vi "Manager QueryPlugin.vi"(6 "contextId":T1, 8 "error in":errorcluster, 9 "timeout (ms)":i32=-1, 10 "Request Data":T17, 11 "gRPC ID":T1) -> (0 "error out":errorcluster, 2 "Response Data":T2, 3 "gRPC ID out":T1)   [LabVIEW 2021, in "CIF_Manager_client.lvlib"]
uses:
  CIF_Manager_client.lvlib
  <vilib>/gRPC/LabVIEW gRPC Library/Shared/grpcId.ctl
  RPC Messages/cif_manager_QueryPluginRequest.ctl
  RPC Messages/cif_manager_QueryPluginResponse.ctl
  RPC Messages/cif_manager_PluginInfo.ctl
  RPC Messages/cif_common_ShortVersion.ctl
  RPC Messages/cif_management_common_PluginStatusData.ctl
  RPC Messages/cif_management_common_PluginStatusData_PluginState.ctl
  RPC Messages/cif_management_common_TimingStatistics.ctl
  RPC Messages/cif_common_TimingStats.ctl
  RPC Messages/cif_management_common_FifoStatistics.ctl
  RPC Messages/cif_management_common_Error.ctl
  RPC Messages/cif_management_common_MonitorDoubles.ctl
  RPC Messages/cif_management_common_MonitorU64.ctl
  RPC Messages/cif_management_common_MonitorI64.ctl
  RPC Messages/cif_management_common_LoaderInfo.ctl
  RPC Messages/cif_management_common_LoaderType.ctl
  RPC Messages/cif_common_Status.ctl
  RPC Messages/cif_manager_QueryPluginResponse_Flat.ctl
  RPC Messages/cif_manager_PluginInfo_Flat.ctl
  RPC Messages/cif_common_ShortVersion_Flat.ctl
  RPC Messages/cif_management_common_PluginStatusData_Flat.ctl
  RPC Messages/cif_management_common_TimingStatistics_Flat.ctl
  RPC Messages/cif_common_TimingStats_Flat.ctl
  RPC Messages/cif_management_common_FifoStatistics_Flat.ctl
  RPC Messages/cif_management_common_Error_Flat.ctl
  RPC Messages/cif_management_common_MonitorDoubles_Flat.ctl
  RPC Messages/cif_management_common_MonitorU64_Flat.ctl
  RPC Messages/cif_management_common_MonitorI64_Flat.ctl
  RPC Messages/cif_management_common_LoaderInfo_Flat.ctl
  RPC Messages/cif_common_Status_Flat.ctl
  14035477-4c25-4107-8ed5-d0c4ef420ce5.vi
  <vilib>/gRPC/LabVIEW gRPC Library/Shared/TranslateGrpcError.vi
  <vilib>/gRPC/LabVIEW gRPC Library/Shared/Wait On Occurrence.vi
  RPC Messages/FlatToRichcif_manager_PluginInfo.vi
  RPC Messages/FlatToRichcif_common_Status.vi
  <vilib>/gRPC/LabVIEW gRPC Library/Shared/Is Feature Enabled.vi
  RPC Messages/FlatToRichcif_common_ShortVersion.vi
  RPC Messages/FlatToRichcif_management_common_PluginStatusData.vi
  RPC Messages/FlatToRichcif_management_common_LoaderInfo.vi
  RPC Messages/FlatToRichcif_management_common_TimingStatistics.vi
  RPC Messages/FlatToRichcif_management_common_FifoStatistics.vi
  RPC Messages/FlatToRichcif_management_common_Error.vi
  RPC Messages/FlatToRichcif_management_common_MonitorDoubles.vi
  RPC Messages/FlatToRichcif_management_common_MonitorU64.vi
  RPC Messages/FlatToRichcif_management_common_MonitorI64.vi
  RPC Messages/FlatToRichcif_common_TimingStats.vi
  <vilib>/gRPC/LabVIEW gRPC Library/Server API/Server/Get Server DLL Path.vi
  <vilib>/Utility/error.llb/Error Cluster From Error Code.vi
  <vilib>/gRPC/LabVIEW gRPC Library/grpc-lvsupport-release.lvlib
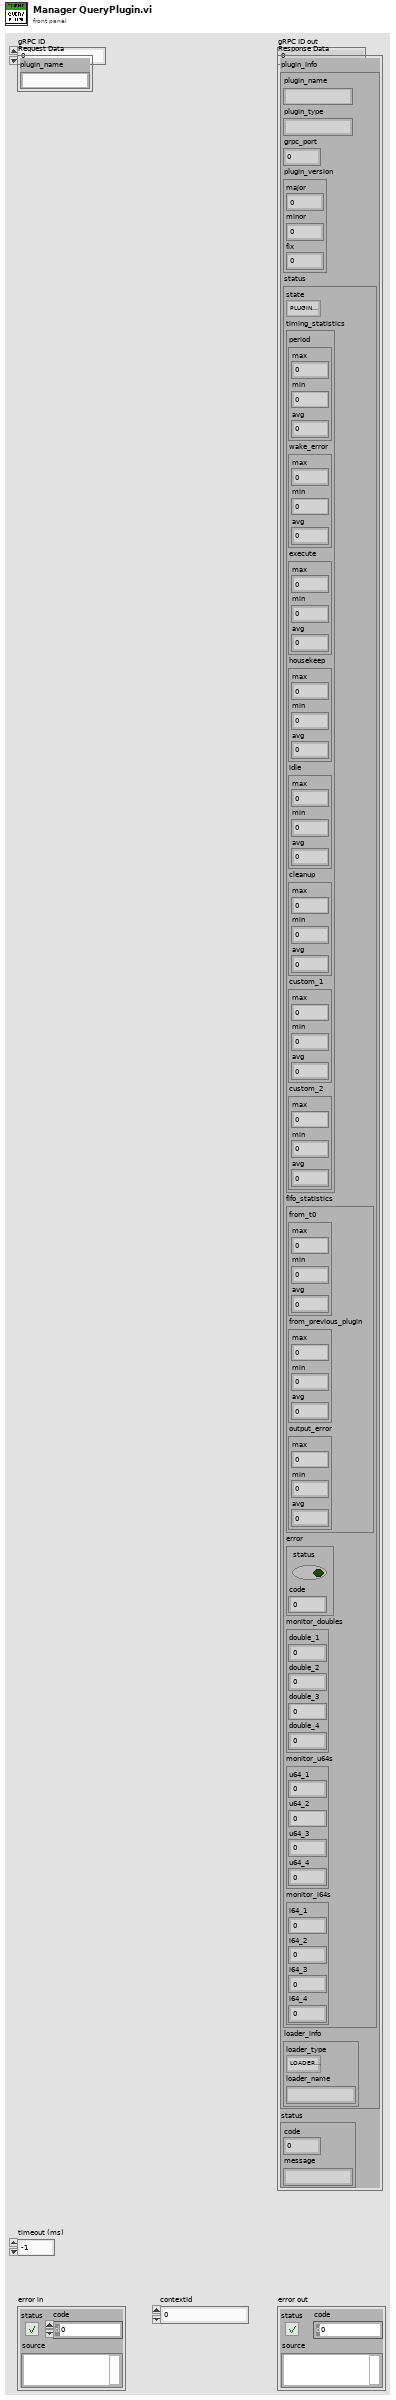
[diagram p1: front panel]
types:
  T1 = typedef "grpc-lvsupport-release.lvlib/grpcId.ctl" = u64
  T2 = typedef "CIF_Manager_client.lvlib/cif_manager_QueryPluginResponse.ctl" = cluster{"plugin_info":T3, "status":T16}
  T3 = typedef "CIF_Manager_client.lvlib/cif_manager_PluginInfo.ctl" = cluster{"plugin_name":string, "plugin_type":string, "grpc_port":i32, "plugin_version":T4, "status":T5, "loader_info":T14}
  T4 = typedef "CIF_Manager_client.lvlib/cif_common_ShortVersion.ctl" = cluster{"major":u32, "minor":u32, "fix":u32}
  T5 = typedef "CIF_Manager_client.lvlib/cif_management_common_PluginStatusData.ctl" = cluster{"state":T6, "timing_statistics":T7, "fifo_statistics":T9, "error":T10, "monitor_doubles":T11, "monitor_u64s":T12, "monitor_i64s":T13}
  T6 = typedef "CIF_Manager_client.lvlib/cif_management_common_PluginStatusData_PluginState.ctl" = enum32{"PLUGINSTATE_UNKNOWN", "PLUGINSTATE_CREATING", "PLUGINSTATE_LISTENING", "PLUGINSTATE_RUNNING", "PLUGINSTATE_CLEANINGUP", "PLUGINSTATE_DESTROYING"}
  T7 = typedef "CIF_Manager_client.lvlib/cif_management_common_TimingStatistics.ctl" = cluster{"period":T8, "wake_error":T8, "execute":T8, "housekeep":T8, "idle":T8, "cleanup":T8, "custom_1":T8, "custom_2":T8}
  T8 = typedef "CIF_Manager_client.lvlib/cif_common_TimingStats.ctl" = cluster{"max":i64, "min":i64, "avg":dbl}
  T9 = typedef "CIF_Manager_client.lvlib/cif_management_common_FifoStatistics.ctl" = cluster{"from_t0":T8, "from_previous_plugin":T8, "output_error":T8}
  T10 = typedef "CIF_Manager_client.lvlib/cif_management_common_Error.ctl" = cluster{"status":bool, "code":i32}
  T11 = typedef "CIF_Manager_client.lvlib/cif_management_common_MonitorDoubles.ctl" = cluster{"double_1":dbl, "double_2":dbl, "double_3":dbl, "double_4":dbl}
  T12 = typedef "CIF_Manager_client.lvlib/cif_management_common_MonitorU64.ctl" = cluster{"u64_1":u64, "u64_2":u64, "u64_3":u64, "u64_4":u64}
  T13 = typedef "CIF_Manager_client.lvlib/cif_management_common_MonitorI64.ctl" = cluster{"i64_1":i64, "i64_2":i64, "i64_3":i64, "i64_4":i64}
  T14 = typedef "CIF_Manager_client.lvlib/cif_management_common_LoaderInfo.ctl" = cluster{"loader_type":T15, "loader_name":string}
  T15 = typedef "CIF_Manager_client.lvlib/cif_management_common_LoaderType.ctl" = enum32{"LOADERTYPE_UNKNOWN", "LOADERTYPE_LABVIEW"}
  T16 = typedef "CIF_Manager_client.lvlib/cif_common_Status.ctl" = cluster{"code":i32, "message":string}
  T17 = typedef "CIF_Manager_client.lvlib/cif_manager_QueryPluginRequest.ctl" = cluster{"plugin_name":string}
  T18 = typedef "CIF_Manager_client.lvlib/cif_manager_QueryPluginResponse_Flat.ctl" = cluster{"plugin_info":T19, "status":T30}
  T19 = typedef "CIF_Manager_client.lvlib/cif_manager_PluginInfo_Flat.ctl" = cluster{"plugin_name":string, "plugin_type":string, "grpc_port":i32, "plugin_version":T20, "status":T21, "loader_info":T29}
  T20 = typedef "CIF_Manager_client.lvlib/cif_common_ShortVersion_Flat.ctl" = cluster{"major":u32, "minor":u32, "fix":u32}
  T21 = typedef "CIF_Manager_client.lvlib/cif_management_common_PluginStatusData_Flat.ctl" = cluster{"state":T6, "timing_statistics":T22, "fifo_statistics":T24, "error":T25, "monitor_doubles":T26, "monitor_u64s":T27, "monitor_i64s":T28}
  T22 = typedef "CIF_Manager_client.lvlib/cif_management_common_TimingStatistics_Flat.ctl" = cluster{"period":T23, "wake_error":T23, "execute":T23, "housekeep":T23, "idle":T23, "cleanup":T23, "custom_1":T23, "custom_2":T23}
  T23 = typedef "CIF_Manager_client.lvlib/cif_common_TimingStats_Flat.ctl" = cluster{"max":i64, "min":i64, "avg":dbl}
  T24 = typedef "CIF_Manager_client.lvlib/cif_management_common_FifoStatistics_Flat.ctl" = cluster{"from_t0":T23, "from_previous_plugin":T23, "output_error":T23}
  T25 = typedef "CIF_Manager_client.lvlib/cif_management_common_Error_Flat.ctl" = cluster{"status":bool, "code":i32}
  T26 = typedef "CIF_Manager_client.lvlib/cif_management_common_MonitorDoubles_Flat.ctl" = cluster{"double_1":dbl, "double_2":dbl, "double_3":dbl, "double_4":dbl}
  T27 = typedef "CIF_Manager_client.lvlib/cif_management_common_MonitorU64_Flat.ctl" = cluster{"u64_1":u64, "u64_2":u64, "u64_3":u64, "u64_4":u64}
  T28 = typedef "CIF_Manager_client.lvlib/cif_management_common_MonitorI64_Flat.ctl" = cluster{"i64_1":i64, "i64_2":i64, "i64_3":i64, "i64_4":i64}
  T29 = typedef "CIF_Manager_client.lvlib/cif_management_common_LoaderInfo_Flat.ctl" = cluster{"loader_type":T15, "loader_name":string}
  T30 = typedef "CIF_Manager_client.lvlib/cif_common_Status_Flat.ctl" = cluster{"code":i32, "message":string}
  T31 = typedef "CIF_Manager_client.lvlib/cif_manager_QueryPluginRequest_Flat.ctl" = cluster{"plugin_name":string}
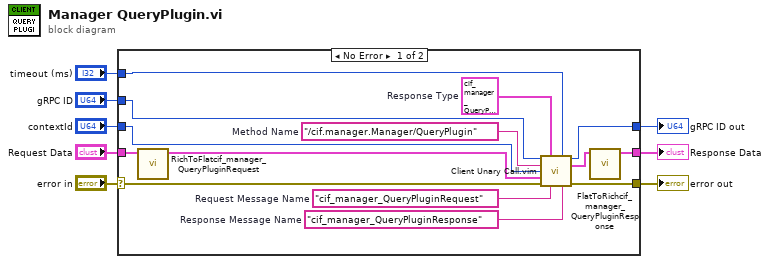
[diagram p0: block diagram]
diagram:
  n1 = case shown="No Error" "error in" {
    selector: "error in" -> [w18 w23]
    tunnel: [w17 w23] -> w7
    tunnel: "gRPC ID" -> [w16 w24]
    tunnel: [w15 w24] -> w5
    tunnel: "Request Data" -> [w12 _]
    tunnel: [w9 _] -> w3
    tunnel: "timeout (ms)" -> [w14 _]
    tunnel: "contextId" -> [w13 _]
    frame No Error {
      w19 = "cif_manager_QueryPluginResponse"  # Response Message Name
      w20 = "cif_manager_QueryPluginRequest"  # Request Message Name
      w21 = T18 {"plugin_info"={"plugin_name"="", "plugin_type"="", "grpc_port"=0, "plugin_version"={"major"=0, "minor"=0, "fix"=0}, "status"={"state"=enum."PLUGINSTATE_UNKNOWN", "timing_statistics"={"period"={"max"=0, "min"=0, "avg"=0.0}, "wake_error"={"max"=0, "min"=0, "avg"=0.0}, "execute"={"max"=0, "min"=0, "avg"=0.0}, "housekeep"={"max"=0, "min"=0, "avg"=0.0}, "idle"={"max"=0, "min"=0, "avg"=0.0}, "cleanup"={"max"=0, "min"=0, "avg"=0.0}, "custom_1"={"max"=0, "min"=0, "avg"=0.0}, "custom_2"={"max"=0, "min"=0, "avg"=0.0}}, "fifo_statistics"={"from_t0"={"max"=0, "min"=0, "avg"=0.0}, "from_previous_plugin"={"max"=0, "min"=0, "avg"=0.0}, "output_error"={"max"=0, "min"=0, "avg"=0.0}}, "error"={"status"=FALSE, "code"=0}, "monitor_doubles"={"double_1"=0.0, "double_2"=0.0, "double_3"=0.0, "double_4"=0.0}, "monitor_u64s"={"u64_1"=0, "u64_2"=0, "u64_3"=0, "u64_4"=0}, "monitor_i64s"={"i64_1"=0, "i64_2"=0, "i64_3"=0, "i64_4"=0}}, "loader_info"={"loader_type"=enum."LOADERTYPE_UNKNOWN", "loader_name"=""}}, "status"={"code"=0, "message"=""}}  # Response Type
      w22 = "/cif.manager.Manager/QueryPlugin"  # Method Name
      n2 = call "RichToFlatcif_manager_QueryPluginRequest.vi"("InputCluster"=w12) -> ("OutputCluster"=w11:T31)  [unwired: 10 in]
      n3 = call "Client Unary Call.vim"("ClientID in"=w16, "Response Type"=w21, "timeout (ms)"=w14, "Method Name"=w22, "contextId"=w13, "Request Data"=w11, "error in"=w18, "Request Message Name"=w20, "Response Message Name"=w19) -> ("ClientID out"=w15:u64, "Response Data"=w10:T18, "error out"=w17:errorcluster)  [unwired: 4 in]
      n4 = call "FlatToRichcif_manager_QueryPluginResponse.vi"("InputCluster"=w10) -> ("OutputCluster"=w9:T2)  [unwired: 10 in]
    }
    frame Error {
    }
  }
  "error out" <- w7
  "gRPC ID out" <- w5
  "Response Data" <- w3
